vi "Set Kasli Name from ID.vi"(8 "error in (no error)":errorcluster, 11 "Kasli Wrapper 2.0 in":refnum<class "Kasli Wrapper 2.0.lvclass">=refnum) -> (0 "error out":errorcluster, 2 "Kasli Name":string, 3 "Kasli Wrapper 2.0 out":refnum<class "Kasli Wrapper 2.0.lvclass">, 4 "Dummy?":bool)   [LabVIEW 2020, in "CIRCUS_uServices.lvlib" / "Kasli Wrapper 2.0.lvlib" / "Kasli Wrapper 2.0.lvclass"]
doc: "This VI interprets the Kasli Name based on the uService ID"
uses:
  Kasli Wrapper 2.0.lvclass
  TALOS/TALOS_PPL.lvlibp
  C:/Users/marco/Documents/GitHub_Lab/CIRCUS/TALOS/TALOS_PPL.lvlibp/Father of all uServices/Father of all uServices/Father of all uServices.lvclass
  C:/Users/marco/Documents/GitHub_Lab/CIRCUS/TALOS/TALOS_PPL.lvlibp/Ancestor/Ancestor/Ancestor.lvclass
  C:/Users/marco/Documents/GitHub_Lab/CIRCUS/TALOS/Actor Framework.lvlibp/1abvi3w/vi.lib/ActorFramework/Actor/Actor.lvclass
  C:/Users/marco/Documents/GitHub_Lab/CIRCUS/CIRCUS uServices et al/Kasli Wrapper 2.0/Kasli Wrapper 2.0.lvclass
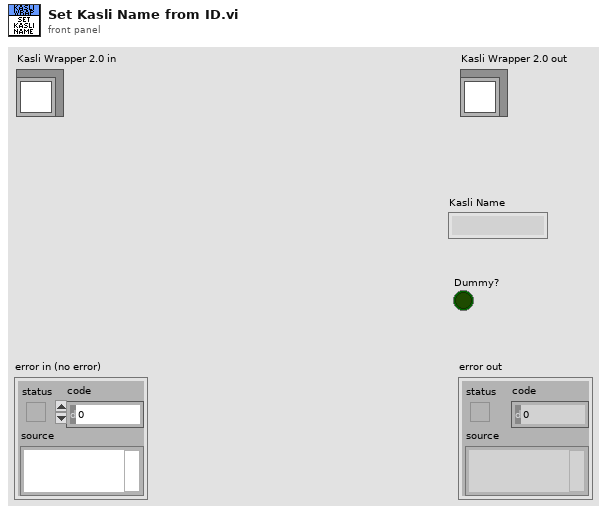
[diagram p1: front panel]
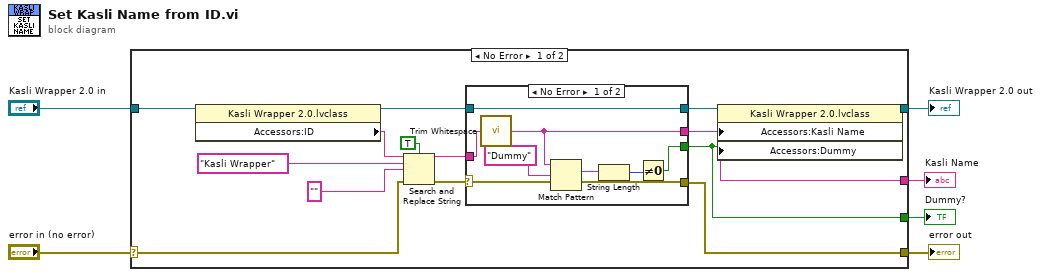
[diagram p0: block diagram]
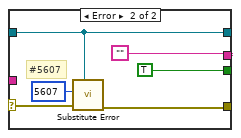
[diagram p2: hidden frame]
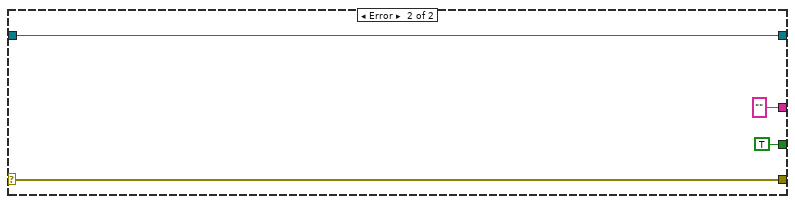
[diagram p3: hidden frame]
diagram:
  n1 = case shown="No Error" "error in (no error)" {
    selector: "error in (no error)" -> [w15 w38]
    tunnel: [w12 w38] -> w5
    tunnel: [w9 w37] -> w3
    tunnel: "Kasli Wrapper 2.0 in" -> [w20 w37]
    tunnel: [w8 "" ("trimmed string")] -> w2
    tunnel: [w7 TRUE ("Dummy")] -> w1
    frame No Error {
      n2 = property class="Kasli Wrapper 2.0.lvclass"(reference=w20) -> (reference out=w11:refnum<class "Kasli Wrapper 2.0.lvclass">, "Accessors:ID"=w19:string)  [unwired: 1 in, 1 out]
      n3 = Search and Replace String(case sensitive?=TRUE ("ignore case? (F)"), input string=w19, search string="Kasli Wrapper", replace string="" ("replace string (\"\")"), error in=w15) -> (result string=w13:string, error out=w14:errorcluster)  [unwired: 3 in, 2 out]
      n4 = case shown="No Error" w14 {
        selector: w14 -> [w27 w34]
        tunnel: w13 -> [w28 _]
        tunnel: [w27 w33] -> w12
        tunnel: [w23 TRUE ("Dummy")] -> w7
        tunnel: [w22 ""] -> w8
        tunnel: w11 -> [w21 w31]
        tunnel: [w21 w31] -> w10
        frame No Error {
          n5 = call <vilib>:"Trim Whitespace.vi"("string"=w28) -> ("trimmed string"=w22:string)  [unwired: 1 in]
          n6 = Match Pattern(string=w22, regular expression="Dummy") -> (match substring=w25:string)  [unwired: 1 in, 3 out]
          n7 = String Length(string=w25) -> (length=w24:i32)
          n8 = Not Equal To 0?(x=w24) -> (x != 0?=w23:bool)
        }
        frame Error {
          # "#5607"
          n9 = call "Substitute Error.vi"("LabVIEW Object"=w31, "error in (no error)"=w34, "Error Code"=5607) -> ("error out"=w33:errorcluster)  [unwired: 8 in]
        }
      }
      n10 = property class="Kasli Wrapper 2.0.lvclass"(reference=w10, "Accessors:Kasli Name"=w8, "Accessors:Dummy"=w7) -> (reference out=w9:refnum<class "Kasli Wrapper 2.0.lvclass">)  [unwired: 1 in, 1 out]
    }
    frame Error {
    }
  }
  "error out" <- w5
  "Kasli Wrapper 2.0 out" <- w3
  "Kasli Name" <- w2
  "Dummy?" <- w1
